vi "Get Ping Message And Reply (SubVI).vi"(0 "input cluster":T1) -> (1 "Consumer out":refnum<class "Queue.lvclass">, 2 "error out":errorcluster)   [LabVIEW 2016]
uses:
  <vilib>/Distrio/LabbitMQ/Queue/Queue.lvclass
  <vilib>/Distrio/LabbitMQ/Exchange/Exchange.lvclass
  <vilib>/Utility/error.llb/DialogType.ctl
  C:/Program Files (x86)/National Instruments/LabVIEW 2016/vi.lib/Distrio/LabbitMQ/RabbitMQ.Client.dll
  Program Files (x86)/National Instruments/LabVIEW 2016/vi.lib/Distrio/LabbitMQ/RabbitMQ.Client.dll
panel:
  in  "stop":bool
  in  "Log":refnum<vi>
  out "Log (current)":string
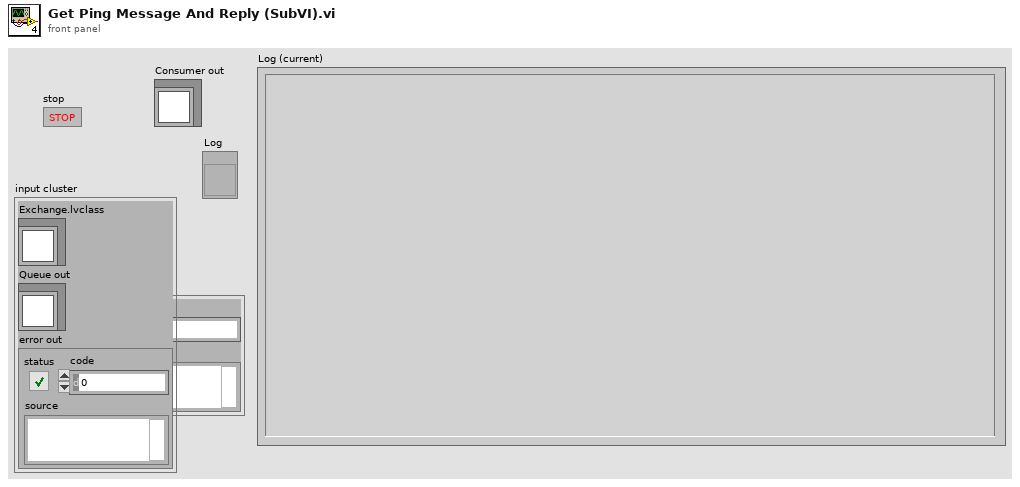
[diagram p1: front panel]
types:
  T1 = cluster{"Exchange.lvclass":refnum<class "Exchange.lvclass">, "Queue out":refnum<class "Queue.lvclass">, "error out":errorcluster}
  T2 = typedef "DialogType.ctl" = u16
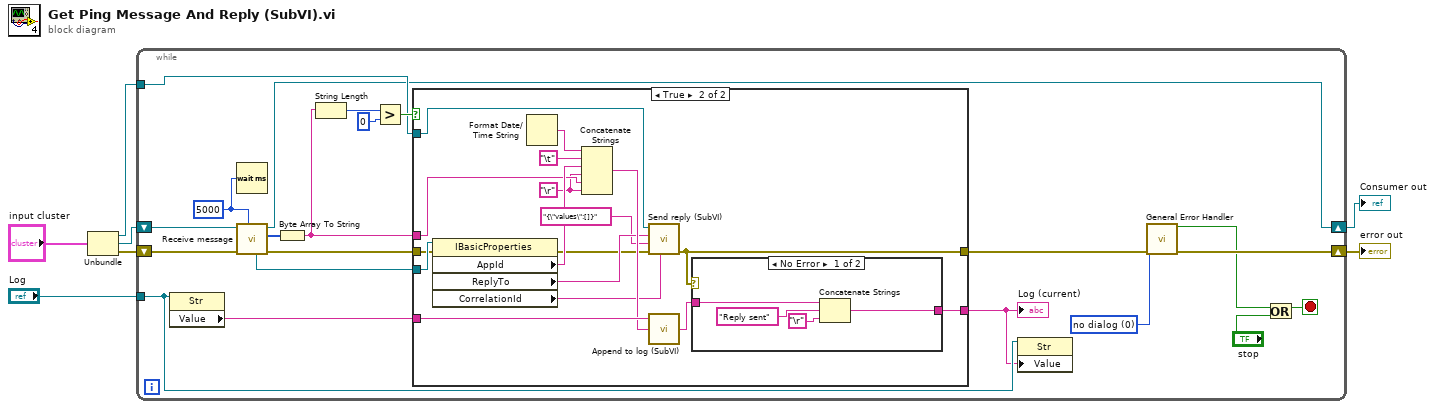
[diagram p0: block diagram]
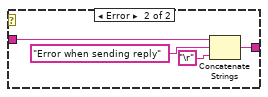
[diagram p3: hidden frame]
diagram:
  n1 = Unbundle("input cluster") -> ("Exchange.lvclass"=w4:refnum<class "Exchange.lvclass">, "Queue out"=w3:refnum<class "Queue.lvclass">, "error out"=w2:errorcluster)
  n2 = while {
    tunnel: w4 -> [w19]
    shift-right: [w11] -> w7
    shift-left: w2 -> [w21]
    tunnel: "Log" -> [w16]
    shift-right: [w14] -> w6
    shift-left: w3 -> [w20]
    stop <- w10 stop-if-true
    w8 = T2 0 items=["no dialog", "OK message", "continue or stop message", "OK message + warnings", "continue/stop + warnings"] ("type of dialog (OK msg:1)")
    w13 = 5000 ("millisecondsTimeout")
    n3 = property class="Str"(reference=w16) -> ("Value"=w17:string)  [unwired: 1 in, 2 out]
    n4 = Wait (ms)(milliseconds to wait=w13) -> ()  [unwired: 1 out]
    n5 = call <vilib>:"Receive message.vi"("millisecondsTimeout"=w13, "error in (no error)"=w21, "Consumer in"=w20) -> ("error out"=w26:errorcluster, "message body"=w28:u8[], "Consumer out"=w14:refnum<class "Queue.lvclass">, "MessageProperties"=w27:refnum<k24>)  [unwired: 3 in, 2 out]
    n6 = Byte Array To String(unsigned byte array=w28) -> (string=w22:string)
    n7 = String Length(string=w22) -> (length=w25:i32)
    n8 = Greater?(x=w25, y=0) -> (0:w23:bool)
    n9 = case shown="True" w23 {
      tunnel: w17 -> [w30 w47]
      tunnel: [w30 w32] -> w15
      tunnel: w27 -> [_ w46]
      tunnel: w22 -> [_ w42]
      tunnel: w26 -> [w29 w40]
      tunnel: [w29 w34] -> w12
      tunnel: w19 -> [_ w39]
      frame False {
      }
      frame True {
        w31 = "\r"
        n10 = property class="IBasicProperties"(reference=w46, error in=w40) -> (error out=w35:errorcluster, "AppId"=w43:string, "ReplyTo"=w38:string, "CorrelationId"=w37:string)  [unwired: 1 out]
        n11 = Format Date/Time String() -> (date/time string=w45:string)  [unwired: 3 in]
        n12 = Concatenate Strings(w45, "\t", w43, w31, w42, w31) -> (w41:string)
        n13 = call "Send reply (SubVI).vi"("Correlation ID"=w37, "error in (no error)"=w35, "reply content"="{\"values\":[]}", "target"=w38, "Exchange.lvclass"=w39) -> ("error out"=w34:errorcluster)  [unwired: 5 in, 1 out]
        n14 = call "Append to log (SubVI).vi"("to append"=w41, "log in"=w47) -> ("log out"=w33:string)  [unwired: 1 in]
        n15 = case shown="No Error" w34 {
          tunnel: w33 -> [w50 w55]
          tunnel: [w48 w52] -> w32
          frame No Error {
            n16 = Concatenate Strings(w50, "Reply sent" ("string"), "\r") -> (w48:string)
          }
          frame Error {
            n17 = Concatenate Strings(w55, "Error when sending reply" ("string"), "\r") -> (w52:string)
          }
        }
      }
    }
    "Log (current)" <- w15
    n18 = property class="Str"(reference=w16, "Value"=w15) -> ()  [unwired: 1 in, 2 out]
    n19 = call <vilib>:"General Error Handler.vi"("type of dialog (OK msg:1)"=w8, "error in (no error)"=w12) -> ("error?"=w9:bool, "error out"=w11:errorcluster)  [unwired: 9 in, 3 out]
    n20 = Or(x=w9, y="stop") -> (x .or. y?=w10:bool)
  }
  "error out" <- w7
  "Consumer out" <- w6
